vi "Calculate Background IA.vi"(6 "Slope":sgl=1.0, 8 "error in":errorcluster, 9 "Wait":i32=5, 10 "Filter":bool, 11 "Cell Data in":refnum<class "PAS Cell Data.lvclass">) -> (0 "error out":errorcluster, 3 "Cell Data out":refnum<class "PAS Cell Data.lvclass">)   [LabVIEW 2014, in "PAS Library.lvlib" / "PAS Cell Data.lvclass"]
doc: "Calculate a running average of the IA when the filter is ON. The running average is pumped into the member <b>IABackground</b>. The first time after a filter switch, there is nothing to average - the background will just be the current value. After this, the background is calculated in a running average as this:\n\nIABackground = (IABackground(avg)*Number_Averaged + IA)/(Number_Averaged+1)\n\nThis will provide a current background of IA for calculating a background corrected absorption over the next sample period."
uses:
  PAS Cell Data.lvclass
  PAS Cell Data.lvclass/PAS Cell Data.ctl
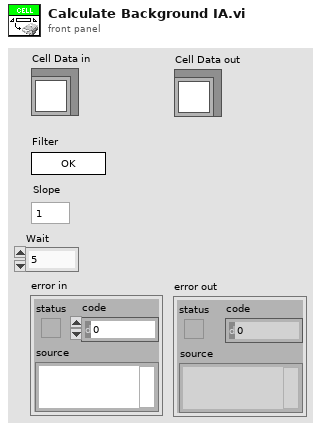
[diagram p1: front panel]
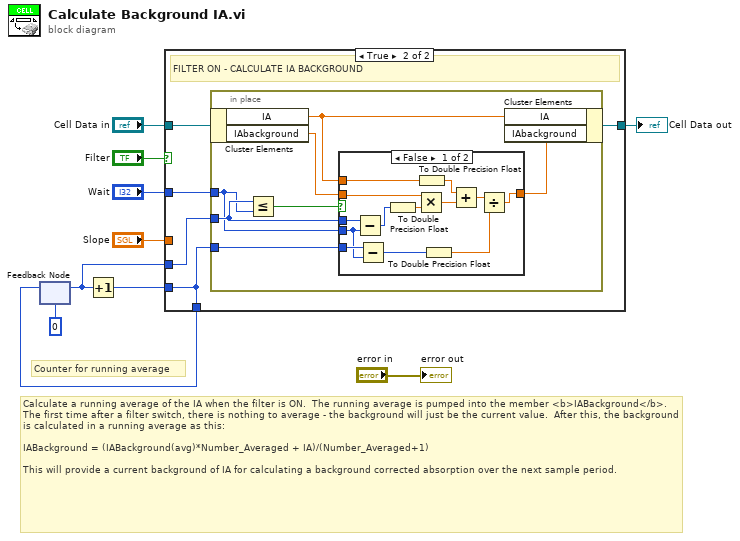
[diagram p0: block diagram]
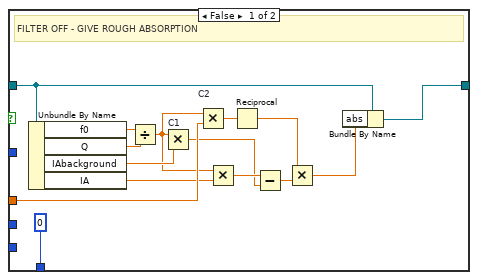
[diagram p2: hidden frame]
diagram:
  # "Calculate a running average of the IA when the filter is ON.  The running average is pumped into the member <b>IABackground</b>.  The first time after a filter switch, there is nothing to average - the background will just be the current value.  After this, the background is calculated in a running average as this:\n\nIABackground = (IABackground(avg)*Number_Averaged + IA)/(Number_Averaged+1)\n\nThis will provide a current background of IA for calculating a background corrected absorption over the next sample period."
  # "Counter for running average"
  n1 = feedback #1(0) -> (w5:i32)
  n2 = Increment(x=w5) -> (x+1=w6:i32)
  n3 = case shown="True" "Filter" {
    tunnel: "Cell Data in" -> [w13 w30]
    tunnel: w6 -> [_ w27]
    tunnel: w5 -> [_ w29]
    tunnel: [0 w27] -> w4
    tunnel: [w12 w28] -> w3
    tunnel: "Slope" -> [w21 _]
    tunnel: "Wait" -> [_ w26]
    frame False {
      # "FILTER OFF - GIVE ROUGH ABSORPTION"
      n4 = Unbundle By Name(w13) -> ("f0"=w24:sgl, "Q"=w23:sgl, "IAbackground"=w22:dbl, "IA"=w19:sgl)
      n5 = Divide(x=w24, y=w23) -> (x/y=w20:sgl)
      n6 = Multiply "C1"(x=w20, y=w22) -> (x*y=w16:dbl)
      n7 = Multiply "C2"(x=w20, y=w21) -> (x*y=w18:sgl)
      n8 = Multiply(x=w20, y=w19) -> (x*y=w17:sgl)
      n9 = Reciprocal(x=w18) -> (1/x=w14:sgl)
      n10 = Subtract(x=w17, y=w16) -> (x-y=w15:dbl)
      n11 = Multiply(x=w14, y=w15) -> (x*y=w11:dbl)
      n12 = Bundle By Name(cluster=w13, "abs"=w11) -> (w12:refnum<class "PAS Cell Data.lvclass">)
    }
    frame True {
      # "FILTER ON - CALCULATE IA BACKGROUND"
      n13 = in-place {
        in-place-border: w29 -> [w33]
        in-place-border: w27 -> [w34]
        in-place-border: w26 -> [w31]
        n14 = in-place-cluster #2(w30) -> ("IA"=w37:sgl, "IAbackground"=w36:dbl)
        n15 = Less Or Equal?(x=w33, y=w31) -> (x <= y?=w32:bool)
        n16 = case shown="False" w32 {
          tunnel: w36 -> [w50 w51]
          tunnel: w37 -> [w43 _]
          tunnel: [w47 w51] -> w35
          tunnel: w33 -> [w42 _]
          tunnel: w34 -> [w40 _]
          tunnel: w31 -> [w39 _]
          frame False {
            n17 = Subtract(x=w42, y=w39) -> (x-y=w41:i32)
            n18 = Subtract(x=w40, y=w39) -> (x-y=w38:i32)
            n19 = To Double Precision Float(number=w41) -> (double precision float=w46:dbl)
            n20 = Multiply(x=w50, y=w46) -> (x*y=w49:dbl)
            n21 = To Double Precision Float(number=w43) -> (double precision float=w44:dbl)
            n22 = To Double Precision Float(number=w38) -> (double precision float=w45:dbl)
            n23 = Add(x=w44, y=w49) -> (x+y=w48:dbl)
            n24 = Divide(x=w48, y=w45) -> (x/y=w47:dbl)
          }
          frame True {
          }
        }
        n25 = in-place-cluster #2("IA"=w37, "IAbackground"=w35) -> (w28:refnum<class "PAS Cell Data.lvclass">)
      }
    }
  }
  "Cell Data out" <- w3
  n26 = feedback-in #1(w4) -> ()
  "error out" <- "error in"
